vi "map_trap_switch_piastre.vi"() -> ()   [LabVIEW 2015]
panel:
  out "output 2":string
  out "command 2":string
  out "Mapping file":string
  in  "Done ?":bool
  in  "KILL":bool
  in  "PAUSE":bool
  in  "RESUME":bool
  in  "QUIT":bool
  in  "Done":bool
  in  "z piastra":bool
  in  "y piastra":bool
  in  "x piastra":bool
  in  "goto y pos":bool
  in  "goto x pos":bool
  in  "End":bool
  in  "zero z - end":bool
  in  "zero x - end":bool
  in  "zero y - end":bool
  in  "positioning done":bool
  out "output":string
  out "command":string
  in  "zero done":bool
  in  "zero z":bool
  in  "zero x":bool
  in  "zero y":bool
  # "Comandi di emergenza"
  # "Posiziono in zero"
  # "Vado sulla piastra \ne azzero"
  # "Vado in posizione\ne parto"
  # "Ritorno a zero"
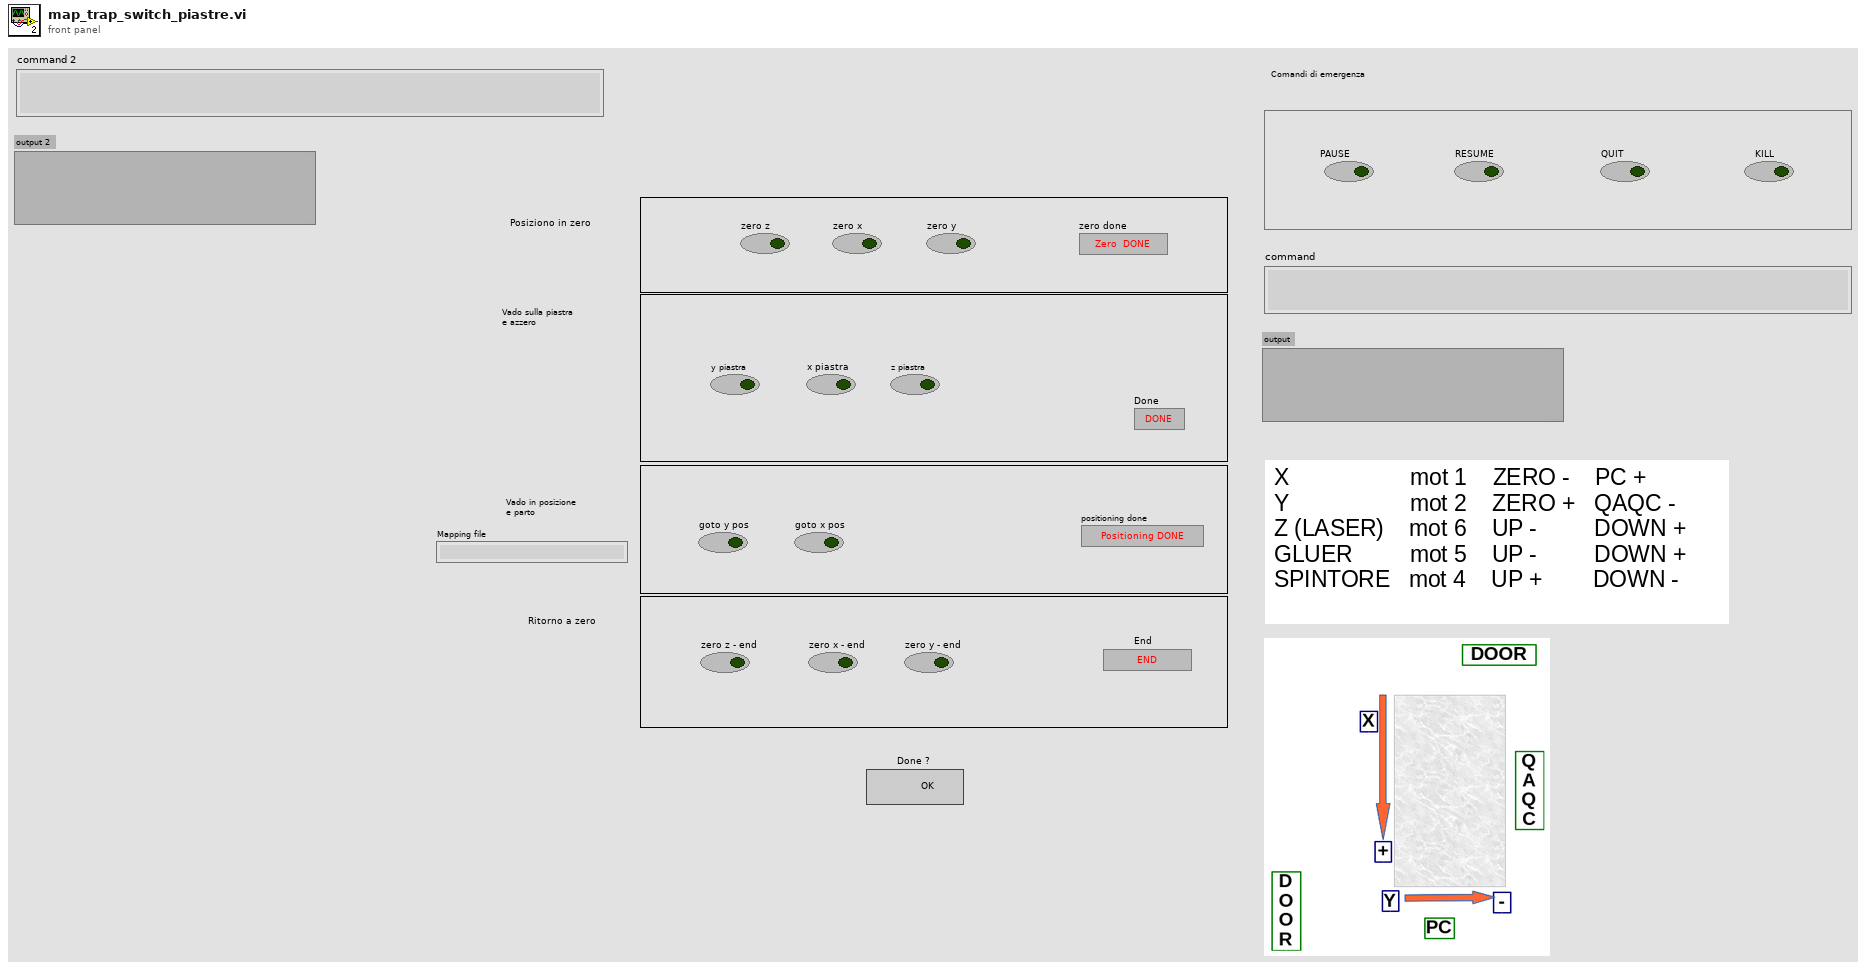
[diagram p1: front panel]
types:
  T1 = enum16{"open", "replace", "create", "open or create", "replace or create", "replace or create with confirmation"}
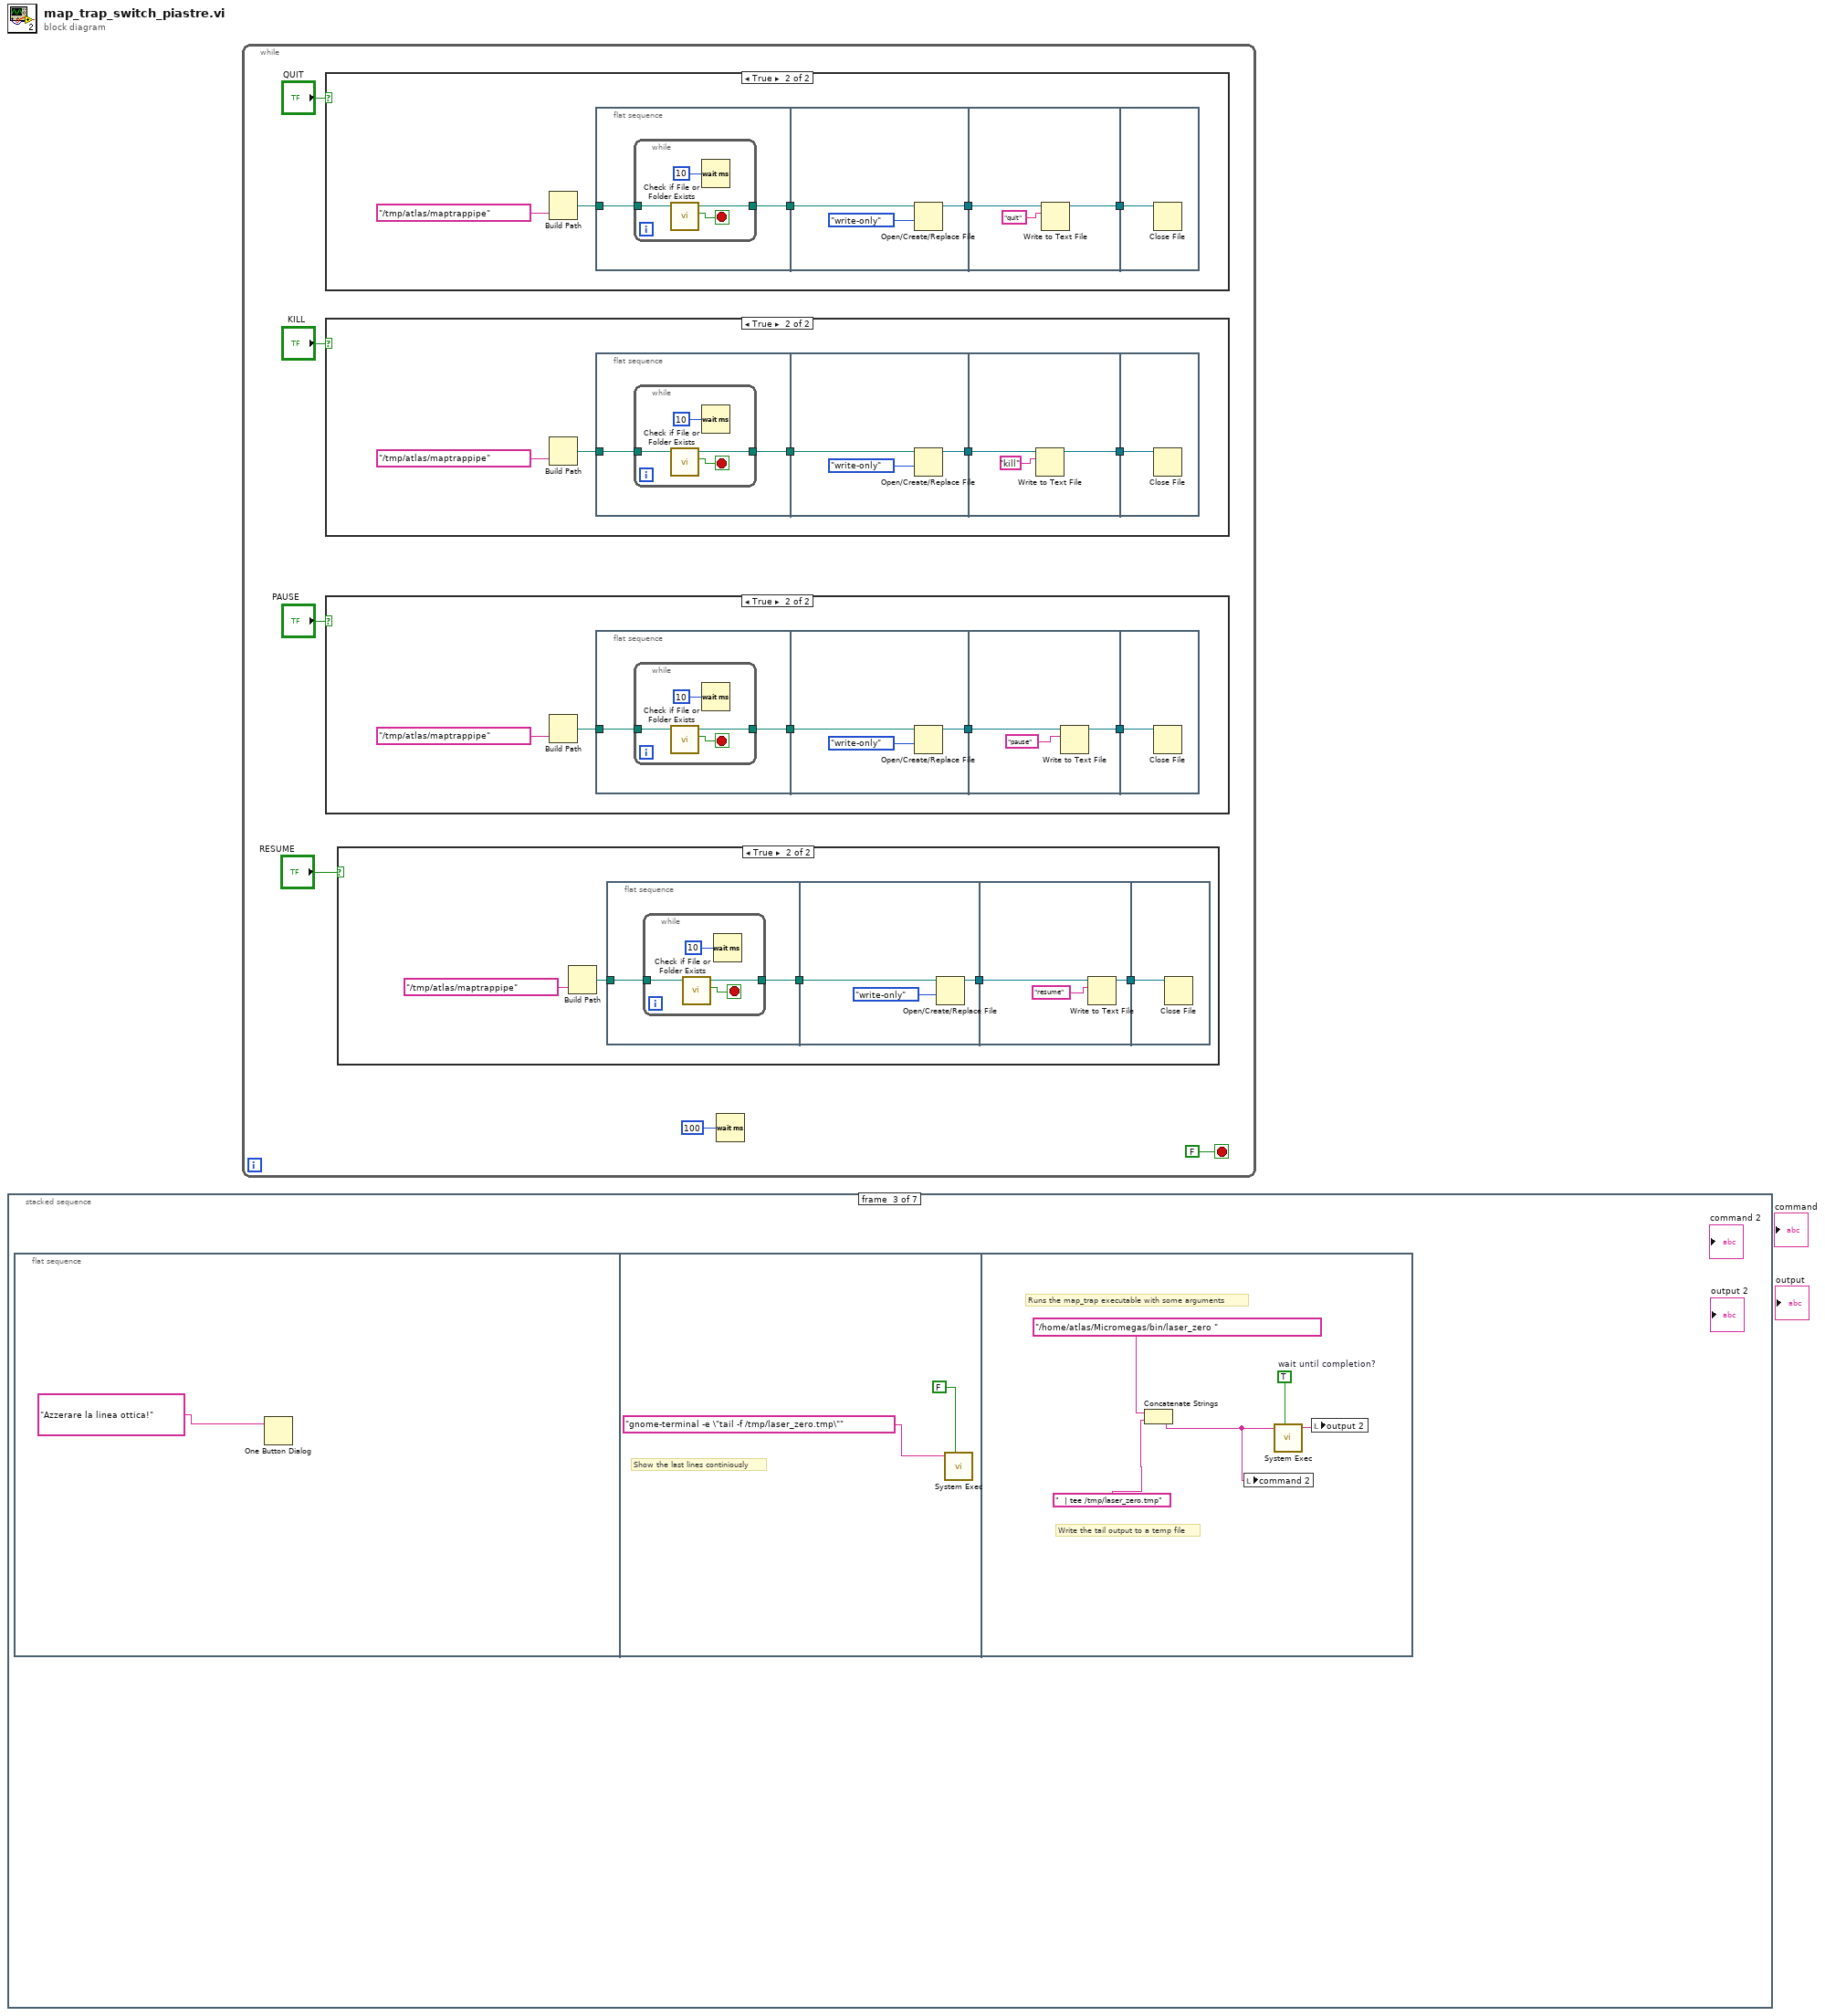
[diagram p0: block diagram]
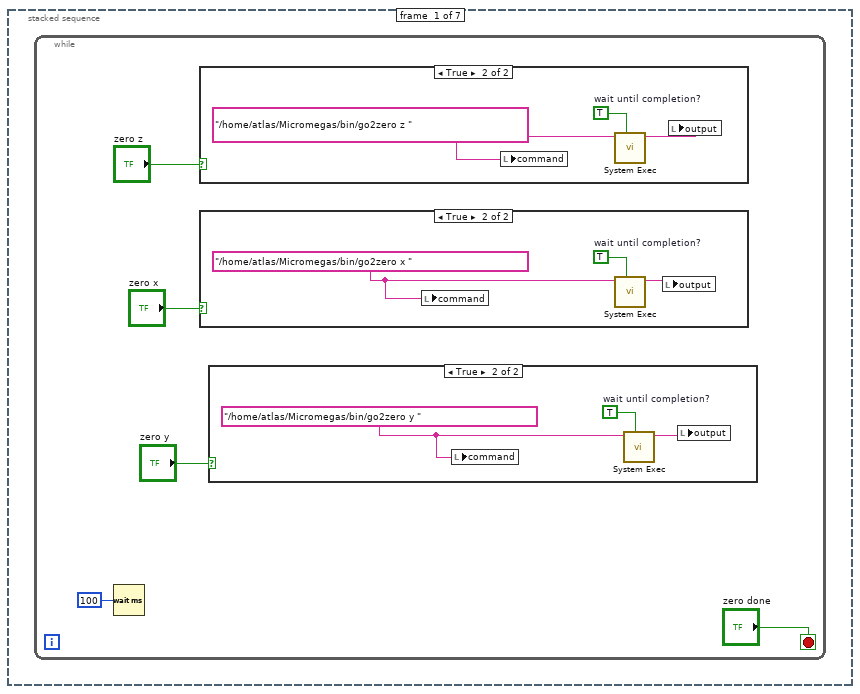
[diagram p6: hidden frame]
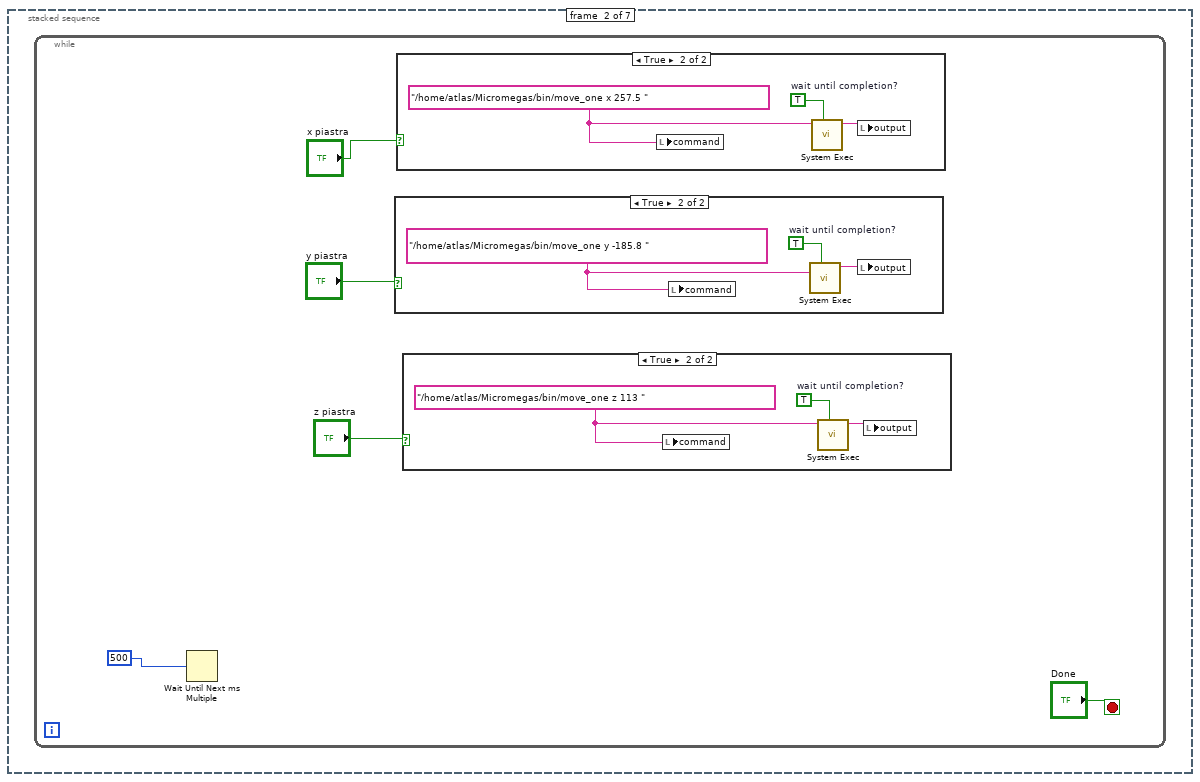
[diagram p10: hidden frame]
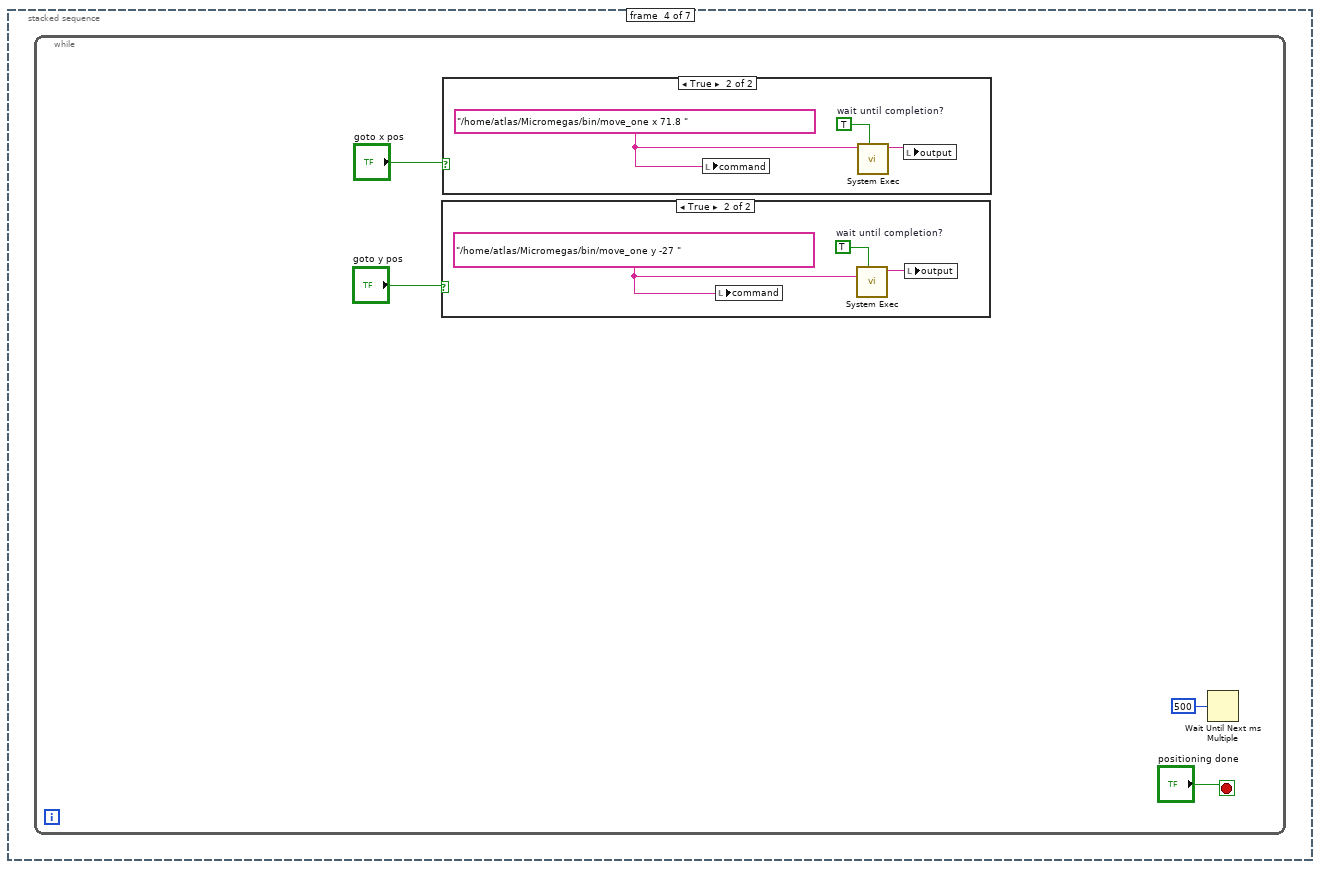
[diagram p14: hidden frame]
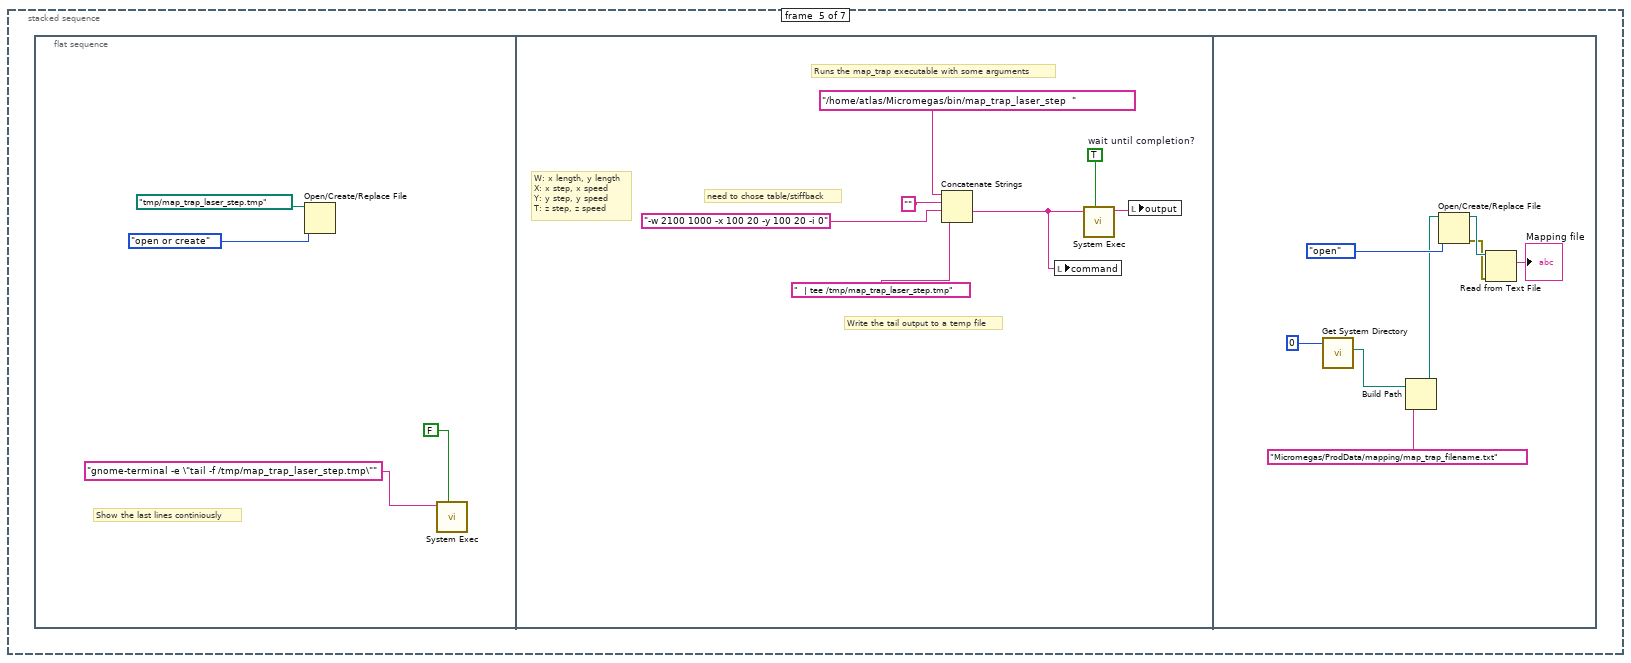
[diagram p17: hidden frame]
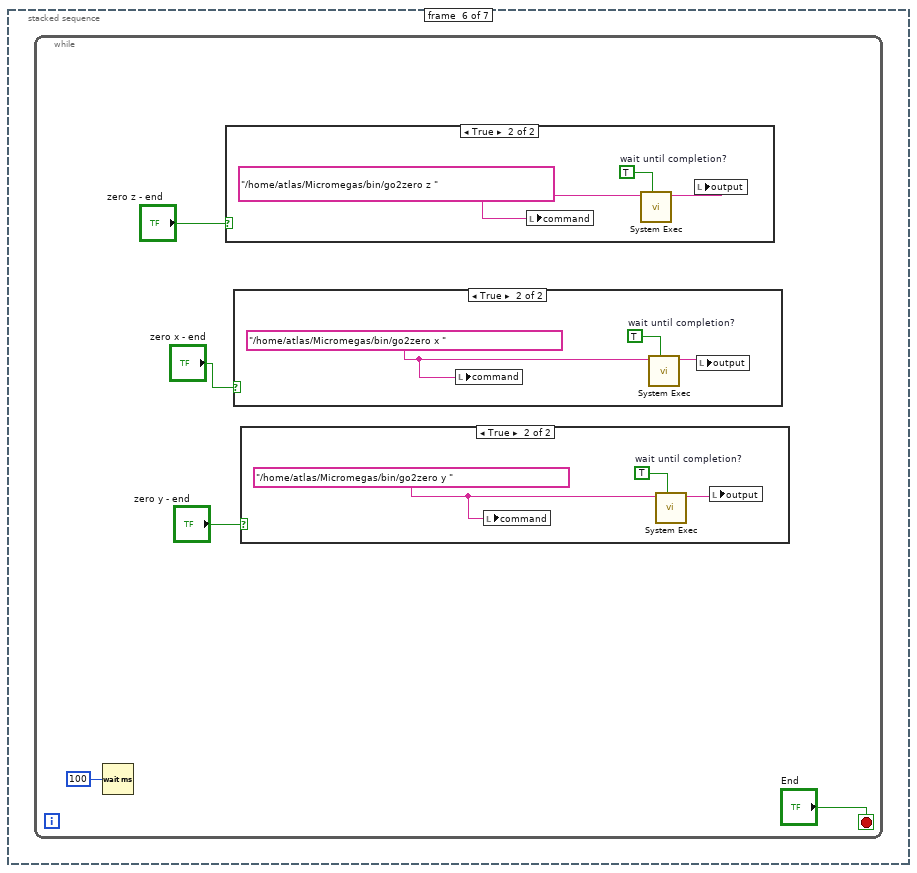
[diagram p18: hidden frame]
diagram:
  n1 = stacked-sequence {
    frame #0 {
      n2 = while {
        stop <- "zero done" stop-if-true
        n3 = Wait (ms)(milliseconds to wait=u32 100) -> ()  [unwired: 1 out]
        n4 = case shown="True" "zero z" {
          frame False {
          }
          frame True {
            w13 = "/home/atlas/Micromegas/bin/go2zero z " ("string")
            w14 = TRUE  # wait until completion?
            n5 = local write "command"(w13) -> ()
            n6 = call <vilib>:"System Exec.vi"("wait until completion? (T)"=w14, "command line"=w13) -> ("standard output"=w12:string)  [unwired: 6 in, 3 out]
            n7 = local write "output"(w12) -> ()
          }
        }
        n8 = case shown="True" "zero x" {
          frame False {
          }
          frame True {
            w10 = "/home/atlas/Micromegas/bin/go2zero x " ("string")
            w11 = TRUE  # wait until completion?
            n9 = local write "command"(w10) -> ()
            n10 = call <vilib>:"System Exec.vi"("wait until completion? (T)"=w11, "command line"=w10) -> ("standard output"=w9:string)  [unwired: 6 in, 3 out]
            n11 = local write "output"(w9) -> ()
          }
        }
        n12 = case shown="True" "zero y" {
          frame False {
          }
          frame True {
            w7 = "/home/atlas/Micromegas/bin/go2zero y " ("string")
            w8 = TRUE  # wait until completion?
            n13 = local write "command"(w7) -> ()
            n14 = call <vilib>:"System Exec.vi"("wait until completion? (T)"=w8, "command line"=w7) -> ("standard output"=w6:string)  [unwired: 6 in, 3 out]
            n15 = local write "output"(w6) -> ()
          }
        }
      }
    }
    frame #1 {
      n16 = while {
        stop <- "Done" stop-if-true
        n17 = Wait Until Next ms Multiple(millisecond multiple=u32 500 ("millisecond timer value")) -> ()  [unwired: 1 out]
        n18 = case shown="True" "y piastra" {
          frame False {
          }
          frame True {
            w23 = "/home/atlas/Micromegas/bin/move_one y -185.8 " ("string")
            w25 = TRUE  # wait until completion?
            n19 = local write "command"(w23) -> ()
            n20 = call <vilib>:"System Exec.vi"("wait until completion? (T)"=w25, "command line"=w23) -> ("standard output"=w24:string)  [unwired: 6 in, 3 out]
            n21 = local write "output"(w24) -> ()
          }
        }
        n22 = case shown="True" "x piastra" {
          frame False {
          }
          frame True {
            w26 = "/home/atlas/Micromegas/bin/move_one x 257.5 " ("string")
            w28 = TRUE  # wait until completion?
            n23 = local write "command"(w26) -> ()
            n24 = call <vilib>:"System Exec.vi"("wait until completion? (T)"=w28, "command line"=w26) -> ("standard output"=w27:string)  [unwired: 6 in, 3 out]
            n25 = local write "output"(w27) -> ()
          }
        }
        n26 = case shown="True" "z piastra" {
          frame False {
          }
          frame True {
            w20 = "/home/atlas/Micromegas/bin/move_one z 113 " ("string")
            w22 = TRUE  # wait until completion?
            n27 = local write "command"(w20) -> ()
            n28 = call <vilib>:"System Exec.vi"("wait until completion? (T)"=w22, "command line"=w20) -> ("standard output"=w21:string)  [unwired: 6 in, 3 out]
            n29 = local write "output"(w21) -> ()
          }
        }
      }
    }
    frame #2 {
      n30 = flat-sequence {
        frame #0 {
          n31 = One Button Dialog(message="Azzerare la linea ottica!") -> ()  [unwired: 1 in, 1 out]
        }
        frame #1 {
          # "Show the last lines continiously"
          n32 = call <vilib>:"System Exec.vi"("wait until completion? (T)"=FALSE, "command line"="gnome-terminal -e \"tail -f /tmp/laser_zero.tmp\"") -> ()  [unwired: 6 in, 4 out]
        }
        frame #2 {
          w36 = TRUE  # wait until completion?
          # "Write the tail output to a temp file"
          # "Runs the map_trap executable with some arguments"
          n33 = Concatenate Strings("/home/atlas/Micromegas/bin/laser_zero " ("string"), "  | tee /tmp/laser_zero.tmp" ("string")) -> (w34:string)
          n34 = local write "command 2"(w34) -> ()
          n35 = call <vilib>:"System Exec.vi"("wait until completion? (T)"=w36, "command line"=w34) -> ("standard output"=w33:string)  [unwired: 6 in, 3 out]
          n36 = local write "output 2"(w33) -> ()
        }
      }
    }
    frame #3 {
      n37 = while {
        stop <- "positioning done" stop-if-true
        n38 = case shown="True" "goto y pos" {
          frame False {
          }
          frame True {
            w41 = "/home/atlas/Micromegas/bin/move_one y -27 " ("string")
            w43 = TRUE  # wait until completion?
            n39 = local write "command"(w41) -> ()
            n40 = call <vilib>:"System Exec.vi"("wait until completion? (T)"=w43, "command line"=w41) -> ("standard output"=w42:string)  [unwired: 6 in, 3 out]
            n41 = local write "output"(w42) -> ()
          }
        }
        n42 = case shown="True" "goto x pos" {
          frame False {
          }
          frame True {
            w44 = "/home/atlas/Micromegas/bin/move_one x 71.8 " ("string")
            w46 = TRUE  # wait until completion?
            n43 = local write "command"(w44) -> ()
            n44 = call <vilib>:"System Exec.vi"("wait until completion? (T)"=w46, "command line"=w44) -> ("standard output"=w45:string)  [unwired: 6 in, 3 out]
            n45 = local write "output"(w45) -> ()
          }
        }
        n46 = Wait Until Next ms Multiple(millisecond multiple=u32 500) -> ()  [unwired: 1 out]
      }
    }
    frame #4 {
      n47 = flat-sequence {
        frame #0 {
          # "Show the last lines continiously"
          n48 = Open/Create/Replace File(file path (use dialog)=path "/tmp/map_trap_laser_step.tmp", operation (0:open)=T1."open or create") -> ()  [unwired: 4 in, 3 out]
          n49 = call <vilib>:"System Exec.vi"("wait until completion? (T)"=FALSE, "command line"="gnome-terminal -e \"tail -f /tmp/map_trap_laser_step.tmp\"") -> ()  [unwired: 6 in, 4 out]
        }
        frame #1 {
          w57 = TRUE  # wait until completion?
          # "need to chose table/stiffback"
          # "Write the tail output to a temp file"
          # "Runs the map_trap executable with some arguments"
          # "W: x length, y length\nX: x step, x speed\nY: y step, y speed\nT: z step, z speed"
          n50 = Concatenate Strings("/home/atlas/Micromegas/bin/map_trap_laser_step  " ("string"), "" ("string"), "-w 2100 1000 -x 100 20 -y 100 20 -i 0" ("string"), "  | tee /tmp/map_trap_laser_step.tmp" ("string")) -> (w52:string)
          n51 = local write "command"(w52) -> ()
          n52 = call <vilib>:"System Exec.vi"("wait until completion? (T)"=w57, "command line"=w52) -> ("standard output"=w51:string)  [unwired: 6 in, 3 out]
          n53 = local write "output"(w51) -> ()
        }
        frame #2 {
          n54 = call <vilib>:"Get System Directory.vi"("system directory type"=0) -> ("system directory"=w59:path)  [unwired: 10 in]
          n55 = Build Path(base path=w59, name or relative path="Micromegas/ProdData/mapping/map_trap_filename.txt") -> (appended path=w58:path)
          n56 = Open/Create/Replace File(file path (use dialog)=w58, operation (0:open)=T1."open") -> (refnum out=w64:refnum<file>, error out=w63:errorcluster)  [unwired: 4 in, 1 out]
          n57 = Read from Text File(file (use dialog)=w64, error in=w63) -> (text=→"Mapping file":string)  [unwired: 2 in, 3 out]
        }
      }
    }
    frame #5 {
      n58 = while {
        stop <- "End" stop-if-true
        n59 = Wait (ms)(milliseconds to wait=u32 100) -> ()  [unwired: 1 out]
        n60 = case shown="True" "zero z - end" {
          frame False {
          }
          frame True {
            w78 = "/home/atlas/Micromegas/bin/go2zero z " ("string")
            w79 = TRUE  # wait until completion?
            n61 = local write "command"(w78) -> ()
            n62 = call <vilib>:"System Exec.vi"("wait until completion? (T)"=w79, "command line"=w78) -> ("standard output"=w77:string)  [unwired: 6 in, 3 out]
            n63 = local write "output"(w77) -> ()
          }
        }
        n64 = case shown="True" "zero x - end" {
          frame False {
          }
          frame True {
            w75 = "/home/atlas/Micromegas/bin/go2zero x " ("string")
            w76 = TRUE  # wait until completion?
            n65 = local write "command"(w75) -> ()
            n66 = call <vilib>:"System Exec.vi"("wait until completion? (T)"=w76, "command line"=w75) -> ("standard output"=w74:string)  [unwired: 6 in, 3 out]
            n67 = local write "output"(w74) -> ()
          }
        }
        n68 = case shown="True" "zero y - end" {
          frame False {
          }
          frame True {
            w72 = "/home/atlas/Micromegas/bin/go2zero y " ("string")
            w73 = TRUE  # wait until completion?
            n69 = local write "command"(w72) -> ()
            n70 = call <vilib>:"System Exec.vi"("wait until completion? (T)"=w73, "command line"=w72) -> ("standard output"=w71:string)  [unwired: 6 in, 3 out]
            n71 = local write "output"(w71) -> ()
          }
        }
      }
    }
    frame #6 {
      n72 = while {
        stop <- "Done ?" stop-if-true
        n73 = case shown="True" "Done ?" {
          frame False {
          }
          frame True {
            n74 = Current VI's Path() -> (path=w82:path)
            n75 = Strip Path(path=w82) -> (name=w83:string)  [unwired: 1 out]
            n76 = call <vilib>:"Close Panel.vi"("VI name"=w83) -> ()  [unwired: 10 in, 1 out]
          }
        }
      }
      n77 = One Button Dialog(message="Per comodita`, rinominare il file (non verra` comunque sovrascritto)") -> ()  [unwired: 1 in, 1 out]
    }
  }
  n78 = while {
    stop <- FALSE stop-if-true
    n79 = case shown="True" "QUIT" {
      frame False {
      }
      frame True {
        n80 = Build Path(name or relative path="/tmp/atlas/maptrappipe" ("string")) -> (appended path=w144:path)  [unwired: 1 in]
        n81 = flat-sequence {
          tunnel: [w150] -> w148
          tunnel: w144 -> [w149]
          tunnel: w148 -> [w157]
          tunnel: [w155] -> w147
          tunnel: w147 -> [w160]
          tunnel: [w159] -> w146
          tunnel: w146 -> [w161]
          frame #0 {
            n82 = while {
              tunnel: [w152] -> w150
              tunnel: w149 -> [w151]
              stop <- w153 stop-if-true
              n83 = call <vilib>:"Check if File or Folder Exists.vi"("path"=w151) -> ("file or folder exists?"=w153:bool, "dup path"=w152:path)  [unwired: 8 in, 1 out]
              n84 = Wait (ms)(milliseconds to wait=u32 10) -> ()  [unwired: 1 out]
            }
          }
          frame #1 {
            n85 = Open/Create/Replace File(file path (use dialog)=w157, access (0:read/write)=enum16{"read/write", "read-only", "write-only"}."write-only") -> (refnum out=w155:refnum<file>)  [unwired: 4 in, 2 out]
          }
          frame #2 {
            n86 = Write to Text File(file (use dialog)=w160, text="quit") -> (refnum out=w159:refnum<file>)  [unwired: 2 in, 2 out]
          }
          frame #3 {
            n87 = Close File(refnum=w161) -> ()  [unwired: 1 in, 2 out]
          }
        }
      }
    }
    n88 = case shown="True" "KILL" {
      frame False {
      }
      frame True {
        n89 = Build Path(name or relative path="/tmp/atlas/maptrappipe" ("string")) -> (appended path=w108:path)  [unwired: 1 in]
        n90 = flat-sequence {
          tunnel: [w114] -> w112
          tunnel: w108 -> [w113]
          tunnel: w112 -> [w121]
          tunnel: [w119] -> w111
          tunnel: w111 -> [w124]
          tunnel: [w123] -> w110
          tunnel: w110 -> [w125]
          frame #0 {
            n91 = while {
              tunnel: [w116] -> w114
              tunnel: w113 -> [w115]
              stop <- w117 stop-if-true
              n92 = call <vilib>:"Check if File or Folder Exists.vi"("path"=w115) -> ("file or folder exists?"=w117:bool, "dup path"=w116:path)  [unwired: 8 in, 1 out]
              n93 = Wait (ms)(milliseconds to wait=u32 10) -> ()  [unwired: 1 out]
            }
          }
          frame #1 {
            n94 = Open/Create/Replace File(file path (use dialog)=w121, access (0:read/write)=enum16{"read/write", "read-only", "write-only"}."write-only") -> (refnum out=w119:refnum<file>)  [unwired: 4 in, 2 out]
          }
          frame #2 {
            n95 = Write to Text File(file (use dialog)=w124, text="kill") -> (refnum out=w123:refnum<file>)  [unwired: 2 in, 2 out]
          }
          frame #3 {
            n96 = Close File(refnum=w125) -> ()  [unwired: 1 in, 2 out]
          }
        }
      }
    }
    n97 = case shown="True" "PAUSE" {
      frame False {
      }
      frame True {
        n98 = Build Path(name or relative path="/tmp/atlas/maptrappipe" ("string")) -> (appended path=w90:path)  [unwired: 1 in]
        n99 = flat-sequence {
          tunnel: [w96] -> w94
          tunnel: w90 -> [w95]
          tunnel: w94 -> [w103]
          tunnel: [w101] -> w93
          tunnel: w93 -> [w106]
          tunnel: [w105] -> w92
          tunnel: w92 -> [w107]
          frame #0 {
            n100 = while {
              tunnel: [w98] -> w96
              tunnel: w95 -> [w97]
              stop <- w99 stop-if-true
              n101 = call <vilib>:"Check if File or Folder Exists.vi"("path"=w97) -> ("file or folder exists?"=w99:bool, "dup path"=w98:path)  [unwired: 8 in, 1 out]
              n102 = Wait (ms)(milliseconds to wait=u32 10) -> ()  [unwired: 1 out]
            }
          }
          frame #1 {
            n103 = Open/Create/Replace File(file path (use dialog)=w103, access (0:read/write)=enum16{"read/write", "read-only", "write-only"}."write-only") -> (refnum out=w101:refnum<file>)  [unwired: 4 in, 2 out]
          }
          frame #2 {
            n104 = Write to Text File(file (use dialog)=w106, text="pause") -> (refnum out=w105:refnum<file>)  [unwired: 2 in, 2 out]
          }
          frame #3 {
            n105 = Close File(refnum=w107) -> ()  [unwired: 1 in, 2 out]
          }
        }
      }
    }
    n106 = case shown="True" "RESUME" {
      frame False {
      }
      frame True {
        n107 = Build Path(name or relative path="/tmp/atlas/maptrappipe" ("string")) -> (appended path=w126:path)  [unwired: 1 in]
        n108 = flat-sequence {
          tunnel: [w132] -> w130
          tunnel: w126 -> [w131]
          tunnel: w130 -> [w139]
          tunnel: [w137] -> w129
          tunnel: w129 -> [w142]
          tunnel: [w141] -> w128
          tunnel: w128 -> [w143]
          frame #0 {
            n109 = while {
              tunnel: [w134] -> w132
              tunnel: w131 -> [w133]
              stop <- w135 stop-if-true
              n110 = call <vilib>:"Check if File or Folder Exists.vi"("path"=w133) -> ("file or folder exists?"=w135:bool, "dup path"=w134:path)  [unwired: 8 in, 1 out]
              n111 = Wait (ms)(milliseconds to wait=u32 10) -> ()  [unwired: 1 out]
            }
          }
          frame #1 {
            n112 = Open/Create/Replace File(file path (use dialog)=w139, access (0:read/write)=enum16{"read/write", "read-only", "write-only"}."write-only") -> (refnum out=w137:refnum<file>)  [unwired: 4 in, 2 out]
          }
          frame #2 {
            n113 = Write to Text File(file (use dialog)=w142, text="resume") -> (refnum out=w141:refnum<file>)  [unwired: 2 in, 2 out]
          }
          frame #3 {
            n114 = Close File(refnum=w143) -> ()  [unwired: 1 in, 2 out]
          }
        }
      }
    }
    n115 = Wait (ms)(milliseconds to wait=100) -> ()  [unwired: 1 out]
  }
